vi "Parse State.vi"(10 "String with Args":string) -> (2 "State":string)   [LabVIEW 2013]
doc: "This sub-VI parses the state from an input string with optional arguments of the form \"state:args\""
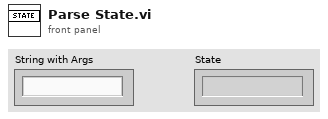
[diagram p1: front panel]
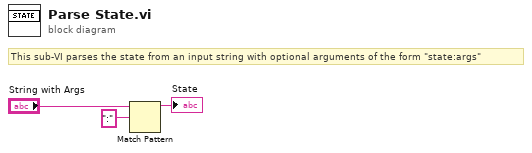
[diagram p0: block diagram]
diagram:
  # "This sub-VI parses the state from an input string with optional arguments of the form \"state:args\""
  n1 = Match Pattern(string="String with Args", regular expression=":") -> (before substring=→"State":string)  [unwired: 1 in, 3 out]
